vi "Get Object Items by Path.vi"(7 "Item Path":string, 8 "error in (no error)":errorcluster, 10 "Object Offset":i32, 11 "JSON":string) -> (0 "error out":errorcluster, 1 "<JSON>":string[](array[string]) caption="Found Items<JSON>", 2 "Names":string[](array[string]))   [LabVIEW 2013, in "JSONtext.lvlib"]
uses:
  JSONtext.lvlib
  support/Unescape JSON string.vi
  support/JSONtext support.lvlib
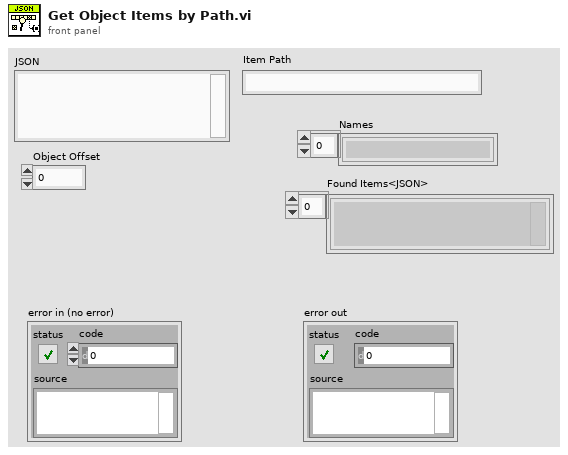
[diagram p1: front panel]
types:
  T1 = typedef "JSONtext.lvlib/Found Items.ctl" = cluster{"Item offset":i32, "Offset past Item":i32, "Name offset":i32, "Offset past Name":i32, "Found":bool, "Empty Object":bool}
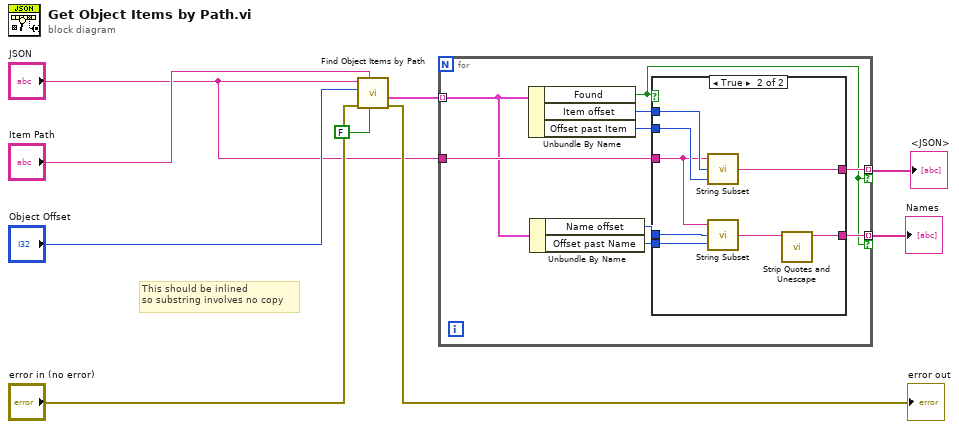
[diagram p0: block diagram]
diagram:
  # "This should be inlined\nso substring involves no copy"
  n1 = call "Find Object Items by Path.vi"("Only return first found"=FALSE, "Path"="Item Path", "error in (no error)"="error in (no error)", "Object Offset"="Object Offset", "JSON"="JSON") -> ("error out"=→"error out":errorcluster, "Items"=w3:T1[])  [unwired: 5 in]
  n2 = for {
    tunnel: "JSON" -> [w18]
    tunnel: [w17] -> w4 mode=indexing if=w10
    tunnel: w3 -> [w14] mode=indexing
    tunnel: [w11] -> w2 mode=indexing if=w10
    n3 = Unbundle By Name(w14) -> ("Found"=w10:bool, "Item offset"=w16:i32, "Offset past Item"=w15:i32)
    n4 = Unbundle By Name(w14) -> ("Name offset"=w12:i32, "Offset past Name"=w13:i32)
    n5 = case shown="True" w10 {
      tunnel: w18 -> [_ w23]
      tunnel: [_ w26] -> w17
      tunnel: w16 -> [_ w25]
      tunnel: w15 -> [_ w24]
      tunnel: w13 -> [_ w22]
      tunnel: w12 -> [_ w21]
      tunnel: [_ w19] -> w11
      frame False {
      }
      frame True {
        n6 = call "String Subset.vi"("Offset past End"=w24, "Start offset"=w25, "JSON"=w23) -> ("substring"=w26:string)  [unwired: 2 in]
        n7 = call "String Subset.vi"("Offset past End"=w22, "Start offset"=w21, "JSON"=w23) -> ("substring"=w20:string)  [unwired: 2 in]
        n8 = call "Strip Quotes and Unescape.vi"("String"=w20) -> ("result string"=w19:string)  [unwired: 9 in, 1 out]
      }
    }
  }
  "<JSON>" <- w4
  "Names" <- w2
